vi "Pulse Switch.vi"(0 "Input Switch":bool, 3 "Time/Loop Time":i32) -> (7 "Pulse Switch":bool, 10 "f":i32)   [LabVIEW 2020]
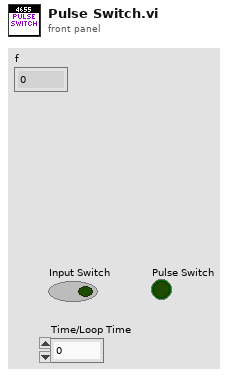
[diagram p1: front panel]
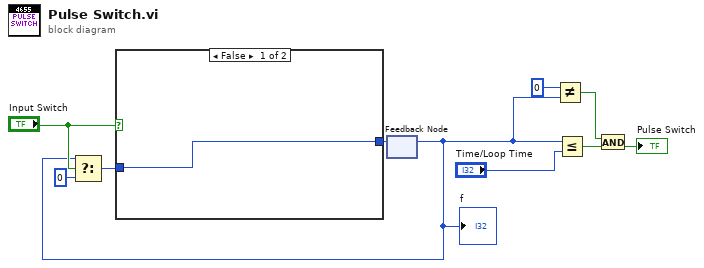
[diagram p0: block diagram]
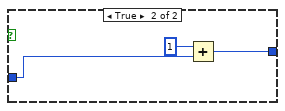
[diagram p2: hidden frame]
diagram:
  n1 = feedback #1() -> (w4:i32)  [unwired: 1 in]
  "f" <- w4
  n2 = Select(t=w4, s="Input Switch", f=0) -> (s? t:f=w8:i32)
  n3 = case shown="False" "Input Switch" {
    tunnel: w8 -> [w11 w14]
    tunnel: [w11 w13] -> w10
    frame False {
    }
    frame True {
      n4 = Add(x=1, y=w14) -> (x+y=w13:i32)
    }
  }
  n5 = feedback-in #1(w10) -> ()
  n6 = Not Equal?(x=0, y=w4) -> (x != y?=w1:bool)
  n7 = Less Or Equal?(x=w4, y="Time/Loop Time") -> (x <= y?=w9:bool)
  n8 = And(x=w1, y=w9) -> (x .and. y?=→"Pulse Switch":bool)
